vi "TREE_Set Symbol.vi"(6 "PicName":string, 7 "Symbol Index":i32, 8 "error in":errorcluster, 9 "Image":T1, 10 "Tag":string, 11 "Tree Ref":refnum<vi>) -> (0 "error out":errorcluster, 3 "Tree Ref":refnum<vi>)   [LabVIEW 2016]
doc: "Set a customize symbol for a item. Notice that all the symbol of items have the same symbol index will change. Set a new symbol index if you want to customize a single item."
uses:
  <vilib>/picture/picture.llb/imagedata.ctl
panel:
  in  "By Image?":bool
  # "Input"
  # "Output"
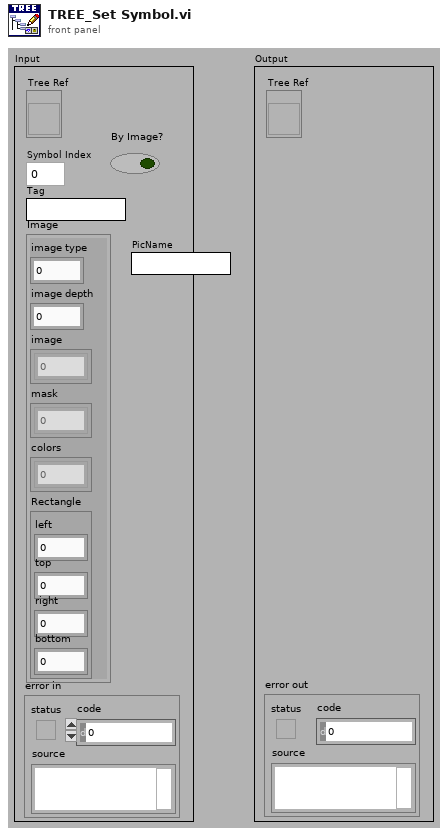
[diagram p1: front panel]
types:
  T1 = typedef "imagedata.ctl" = cluster{"image type":i32, "image depth":i32, "image":u8[], "mask":u8[], "colors":u32[], "Rectangle":cluster{"left":i16, "top":i16, "right":i16, "bottom":i16}}
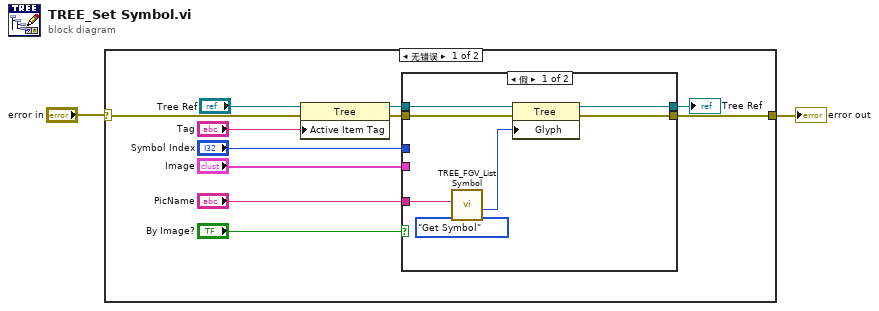
[diagram p0: block diagram]
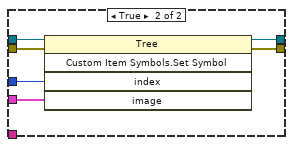
[diagram p2: hidden frame]
diagram:
  n1 = case shown="无错误" "error in" {
    selector: "error in" -> [w6 w27]
    tunnel: [w7 w27] -> w2
    frame No Error {
      n2 = property class="Tree"(reference="Tree Ref", error in=w6, "Active Item Tag"="Tag") -> (reference out=w13:refnum<vi>, error out=w12:errorcluster)
      n3 = case shown="假" "By Image?" {
        tunnel: w13 -> [w20 w26]
        tunnel: w12 -> [w19 w25]
        tunnel: "Symbol Index" -> [_ w24]
        tunnel: [w17 w23] -> w8
        tunnel: [w18 w22] -> w7
        tunnel: "Image" -> [_ w21]
        tunnel: "PicName" -> [w14 _]
        frame False {
          n4 = call "TREE_FGV_List Symbol.vi"("Oper"=enum16{"Initial", "Get Symbol", "Clear"}."Get Symbol", "Picture Name"=w14) -> ("Symbol Index"=w15:i32)  [unwired: 9 in]
          n5 = property class="Tree"(reference=w20, error in=w19, "Glyph"=w15) -> (reference out=w17:refnum<vi>, error out=w18:errorcluster)
        }
        frame True {
          n6 = invoke class="Tree" method="Custom Item Symbols.Set Symbol"(reference=w26, error in=w25, "index"=w24, "image"=w21) -> (reference out=w23:refnum<vi>, error out=w22:errorcluster)  [unwired: 1 in, 3 out]
        }
      }
      "Tree Ref" <- w8
    }
    frame Error {
    }
  }
  "error out" <- w2
